vi "GetTagsByKeyword.vi"(10 "keyword":string, 11 "tags":T1[](array[typedef])) -> (3 "matches":T1[](array[typedef]))   [LabVIEW 2017, in "DeviceModelHelpers.lvlib"]
doc: "Returns all tags that match a particular keyword."
uses:
  <vilib>/addons/InsightCM/Utilities/DeviceModelHelpers/DeviceModelHelpers.lvlib
  <vilib>/addons/InsightCM/MessageBus/Base/controls/Tag.ctl
  <vilib>/addons/InsightCM/MessageBus/Base/controls/KeyValuePair.ctl
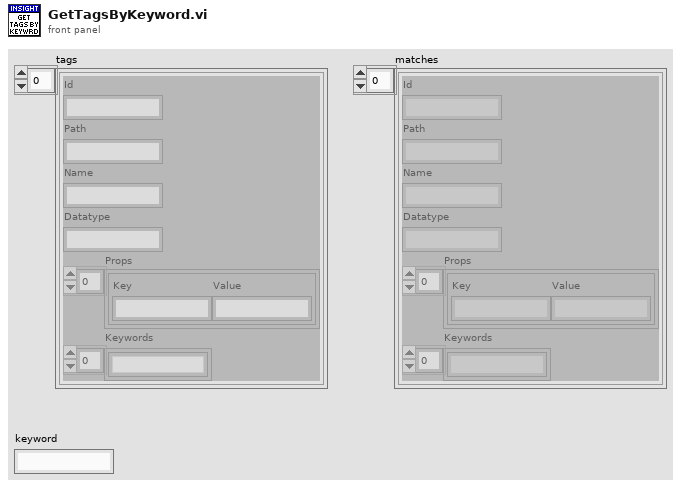
[diagram p1: front panel]
types:
  T1 = typedef "Tag.ctl" = cluster{"Id":string, "Path":string, "Name":string, "Datatype":string, "Props":T2[], "Keywords":string[]}
  T2 = typedef "KeyValuePair.ctl" = cluster{"Key":string, "Value":string}
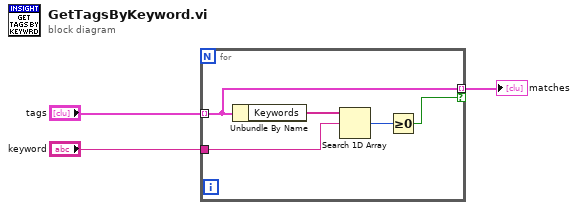
[diagram p0: block diagram]
diagram:
  n1 = for {
    tunnel: "tags" -> [w8] mode=indexing
    tunnel: "keyword" -> [w6]
    tunnel: [w8] -> w1 mode=indexing if=w4
    n2 = Unbundle By Name(w8) -> ("Keywords"=w7:string[])
    n3 = Search 1D Array(1D array=w7, element=w6) -> (index of element=w5:i32)  [unwired: 1 in]
    n4 = Greater Or Equal To 0?(x=w5) -> (x >= 0?=w4:bool)
  }
  "matches" <- w1
